vi "uObserver_Get_Policy_Pub.vi"(8 "error in (no error)":errorcluster, 11 "uObserver in":refnum<class "uObserver.lvclass">) -> (0 "error out":errorcluster, 2 "uStringManipulation":refnum<class "uStringManipulation.lvclass">, 3 "uObserver out":refnum<class "uObserver.lvclass">)   [LabVIEW 2023, in "uLib.lvlib" / "uObserver.lvclass"]
doc: "Allows a child to get the publishing policy that was passed in the by the actor's runtime caller. This may be used to manipulate the policy when executing the registration action."
uses:
  uObserver.lvclass
  uStringManipulation/uStringManipulation/uStringManipulation.lvclass
  uObserver.lvclass/uObserver.ctl
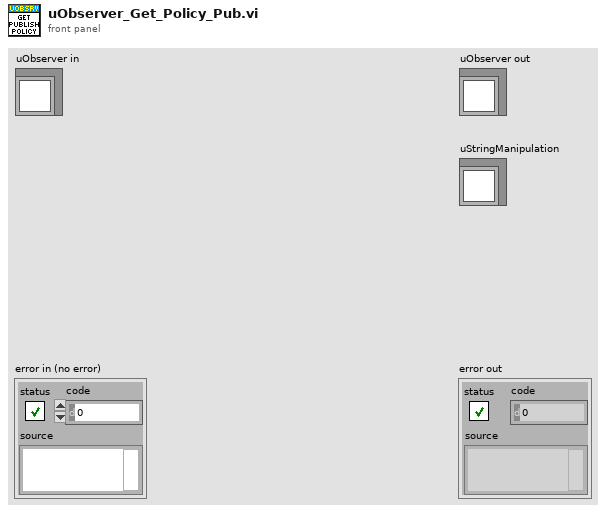
[diagram p1: front panel]
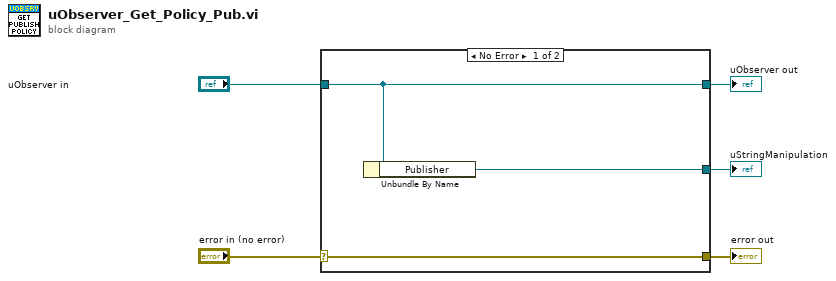
[diagram p0: block diagram]
diagram:
  n1 = case shown="No Error" "error in (no error)" {
    selector: "error in (no error)" -> [w8 w9]
    tunnel: [w8 w9] -> w4
    tunnel: [w7 w10] -> w2
    tunnel: "uObserver in" -> [w7 w10]
    tunnel: [w6 _] -> w1
    frame No Error {
      n2 = Unbundle By Name(w7) -> ("Publisher"=w6:refnum<class "uStringManipulation.lvclass">)
    }
    frame Error {
    }
  }
  "error out" <- w4
  "uObserver out" <- w2
  "uStringManipulation" <- w1
